vi "Inverse Time Curves (Curve Data).vi"(6 "operate time compensation":cluster{"G/Gs":dbl, "compensation [s]":dbl}[](array[cluster]), 8 "error in (no error)":errorcluster, 11 "curve data":T1(array[cluster])) -> (0 "error out":errorcluster, 2 "memory size":u16, 3 "memory initial values":fxp<+,51,51>[](array[numeric]), 4 "actual curve data":cluster{"G/Gs":dbl[], "times [s]":dbl[]})   [LabVIEW 2013, in "NI_EP_Protection.lvlib"]
doc: "Generates memory initial values and memory size, which contain the information of the inverse time curves, for the FPGA Inverse Time Delay VI to use. You can compensate for the processing delay of the input energizing quantity under a specific G/Gs to achieve higher operate time accuracy."
uses:
  <vilib>/addons/Electrical Power/Protection/NI_EP_Protection.lvlib
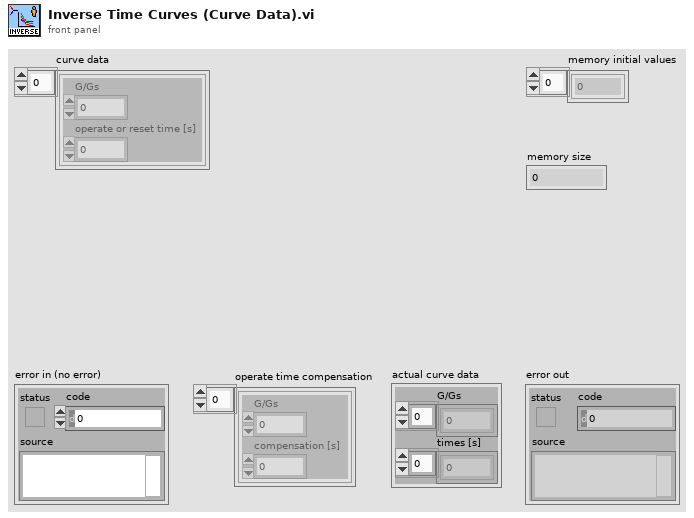
[diagram p1: front panel]
types:
  T1 = cluster{"G/Gs":dbl, "operate or reset time [s]":dbl}[]
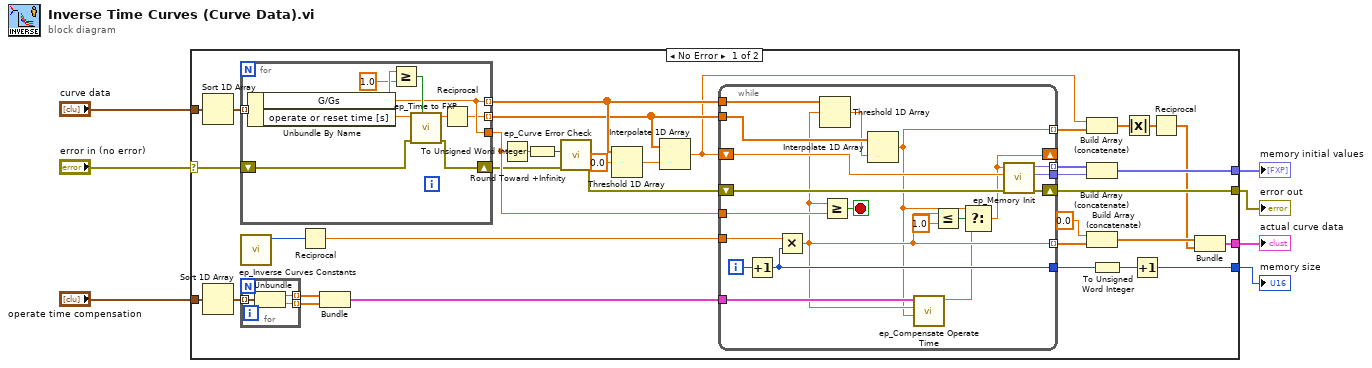
[diagram p0: block diagram]
diagram:
  n1 = case shown="No Error" "error in (no error)" {
    selector: "error in (no error)" -> [w34 w75]
    tunnel: "curve data" -> [w42 _]
    tunnel: [w37 _] -> w5
    tunnel: [w22 _] -> w4
    tunnel: [w18 _] -> w3
    tunnel: [w17 w75] -> w2
    tunnel: "operate time compensation" -> [w12 _]
    frame No Error {
      n2 = Sort 1D Array(array=w42) -> (sorted array=w41:T1)
      n3 = Sort 1D Array(array=w12) -> (sorted array=w11:cluster{"G/Gs":dbl, "compensation [s]":dbl}[])
      n4 = for {
        tunnel: w41 -> [w74] mode=indexing
        tunnel: [w68] -> w32 mode=indexing
        tunnel: [w66] -> w30 mode=indexing
        tunnel: [w68] -> w36
        shift-right: [w70] -> w33
        shift-left: w34 -> [w72]
        n5 = Unbundle By Name(w74) -> ("G/Gs"=w68:dbl, "operate or reset time [s]"=w73:dbl)
        n6 = Greater Or Equal?(x=w68, y=1.0) -> (x >= y?=w69:bool)
        n7 = call <vilib>:"ep_Time to FXP.vi"("operate?"=w69, "error in (no error)"=w72, "time"=w73) -> ("error out"=w70:errorcluster, "time"=w71:dbl)  [unwired: 7 in]
        n8 = Reciprocal(x=w71) -> (1/x=w66:dbl)
      }
      n9 = call <vilib>:"ep_Inverse Curves Constants.vi"() -> ("number of sections in each G/Gs step"=w40:u16)  [unwired: 6 in, 5 out]
      n10 = for {
        tunnel: w11 -> [w45] mode=indexing
        tunnel: [w44] -> w10 mode=indexing
        tunnel: [w43] -> w9 mode=indexing
        n11 = Unbundle(w45) -> ("G/Gs"=w44:dbl, "compensation [s]"=w43:dbl)
      }
      n12 = Reciprocal(x=w40) -> (1/x=w39:dbl)
      n13 = Bundle(w10, w9) -> (w8:cluster{dbl[], dbl[]})  [unwired: 1 in]
      n14 = Round Toward +Infinity(x=w36) -> (ceil(x): smallest int >= x=w14:dbl)
      n15 = To Unsigned Word Integer(number=w14) -> (unsigned 16bit integer=w13:u16)
      n16 = call <vilib>:"ep_Curve Error Check.vi"("error in (no error)"=w33, "GD"=w13) -> ("error out"=w29:errorcluster)  [unwired: 9 in]
      n17 = Threshold 1D Array(2:0.0 ("threshold y"), 3:w32) -> (0:w31:dbl)  [unwired: 1 in]
      n18 = Interpolate 1D Array(1:w31, 2:w30) -> (0:w23:dbl)
      n19 = while {
        tunnel: w32 -> [w65]
        tunnel: w39 -> [w64]
        tunnel: w36 -> [w63]
        tunnel: [w60] -> w38
        tunnel: [w50] -> w25 mode=indexing
        shift-right: [w46] -> _
        shift-left: w23 -> [w57]
        tunnel: w30 -> [w59]
        tunnel: [w56] -> w28 mode=indexing
        tunnel: [w55] -> w27
        tunnel: [w48] -> w24 mode=indexing
        shift-right: [w53] -> w17
        shift-left: w29 -> [w54]
        tunnel: w8 -> [w51]
        i -> [w61]
        stop <- w62 stop-if-true
        n20 = Increment(x=w61) -> (x+1=w60:i32)
        n21 = Multiply(x=w64, y=w60) -> (x*y=w50:dbl)
        n22 = Threshold 1D Array(2:w50, 3:w65) -> (0:w58:dbl)  [unwired: 1 in]
        n23 = Greater Or Equal?(x=w50, y=w63) -> (x >= y?=w62:bool)
        n24 = Interpolate 1D Array(1:w58, 2:w59) -> (0:w48:dbl)
        n25 = call <vilib>:"ep_Compensate Operate Time.vi"("operate time"=w48, "multiples of pickup"=w50, "operate time compensation"=w51) -> ("compensated operate time"=w47:dbl)  [unwired: 8 in]
        n26 = Less Or Equal?(x=w50, y=1.0) -> (x <= y?=w49:bool)
        n27 = Select(t=w48, s=w49, f=w47) -> (s? t:f=w46:dbl)
        n28 = call <vilib>:"ep_Memory Init.vi"("error in (no error)"=w54, "1/previous time"=w57, "1/time"=w46) -> ("error out"=w53:errorcluster, "last memory initial value"=w55:fxp<+,51,51>, "memory initial value"=w56:fxp<+,51,51>)  [unwired: 6 in]
      }
      n29 = Build Array (concatenate)(w23, w24) -> (w20:dbl[])
      n30 = Build Array (concatenate)(w28, w27) -> (w22:fxp<+,51,51>[])
      n31 = Build Array (concatenate)(0.0 ("multiples of pickup"), w25) -> (w19:dbl[])
      n32 = To Unsigned Word Integer(number=w38) -> (unsigned 16bit integer=w35:u16)
      n33 = Absolute Value(x=w20) -> (abs(x)=w21:dbl[])
      n34 = Increment(x=w35) -> (x+1=w37:u16)
      n35 = Reciprocal(x=w21) -> (1/x=w15:dbl[])
      n36 = Bundle(w19, w15) -> (w18:cluster{dbl[], dbl[]})  [unwired: 1 in]
    }
    frame Error {
    }
  }
  "memory initial values" <- w4
  "error out" <- w2
  "memory size" <- w5
  "actual curve data" <- w3
